vi "ElevFF_CalculateVelocityOnly.vi"(10 "Velocity":dbl, 11 "in ELEV_FF":T1 {"Kg" format="%13.5p"; "Ka" format="%13.5p"; "Kv" format="%13.5p"; "Ks" format="%13.5p"}) -> (3 "FeedForward":dbl)   [LabVIEW 2019, in "Trajectory_Library.lvlib"]
doc: "Calculates the feedforward from the gains and velocity setpoint (acceleration is assumed to be zero).\n \nInputs: \n - ElevFF -- The ElevFF data cluster\n - velocity -- The velocity setpoint.\n\nOutputs:\n - feedforward -- The computed feedforward."
uses:
  Trajectory_Library.lvlib
  ELEV_FF.ctl
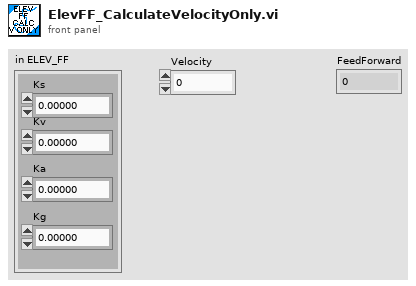
[diagram p1: front panel]
types:
  T1 = typedef "Trajectory_Library.lvlib/ELEV_FF.ctl" = cluster{"Ks":dbl, "Kv":dbl, "Ka":dbl, "Kg":dbl}
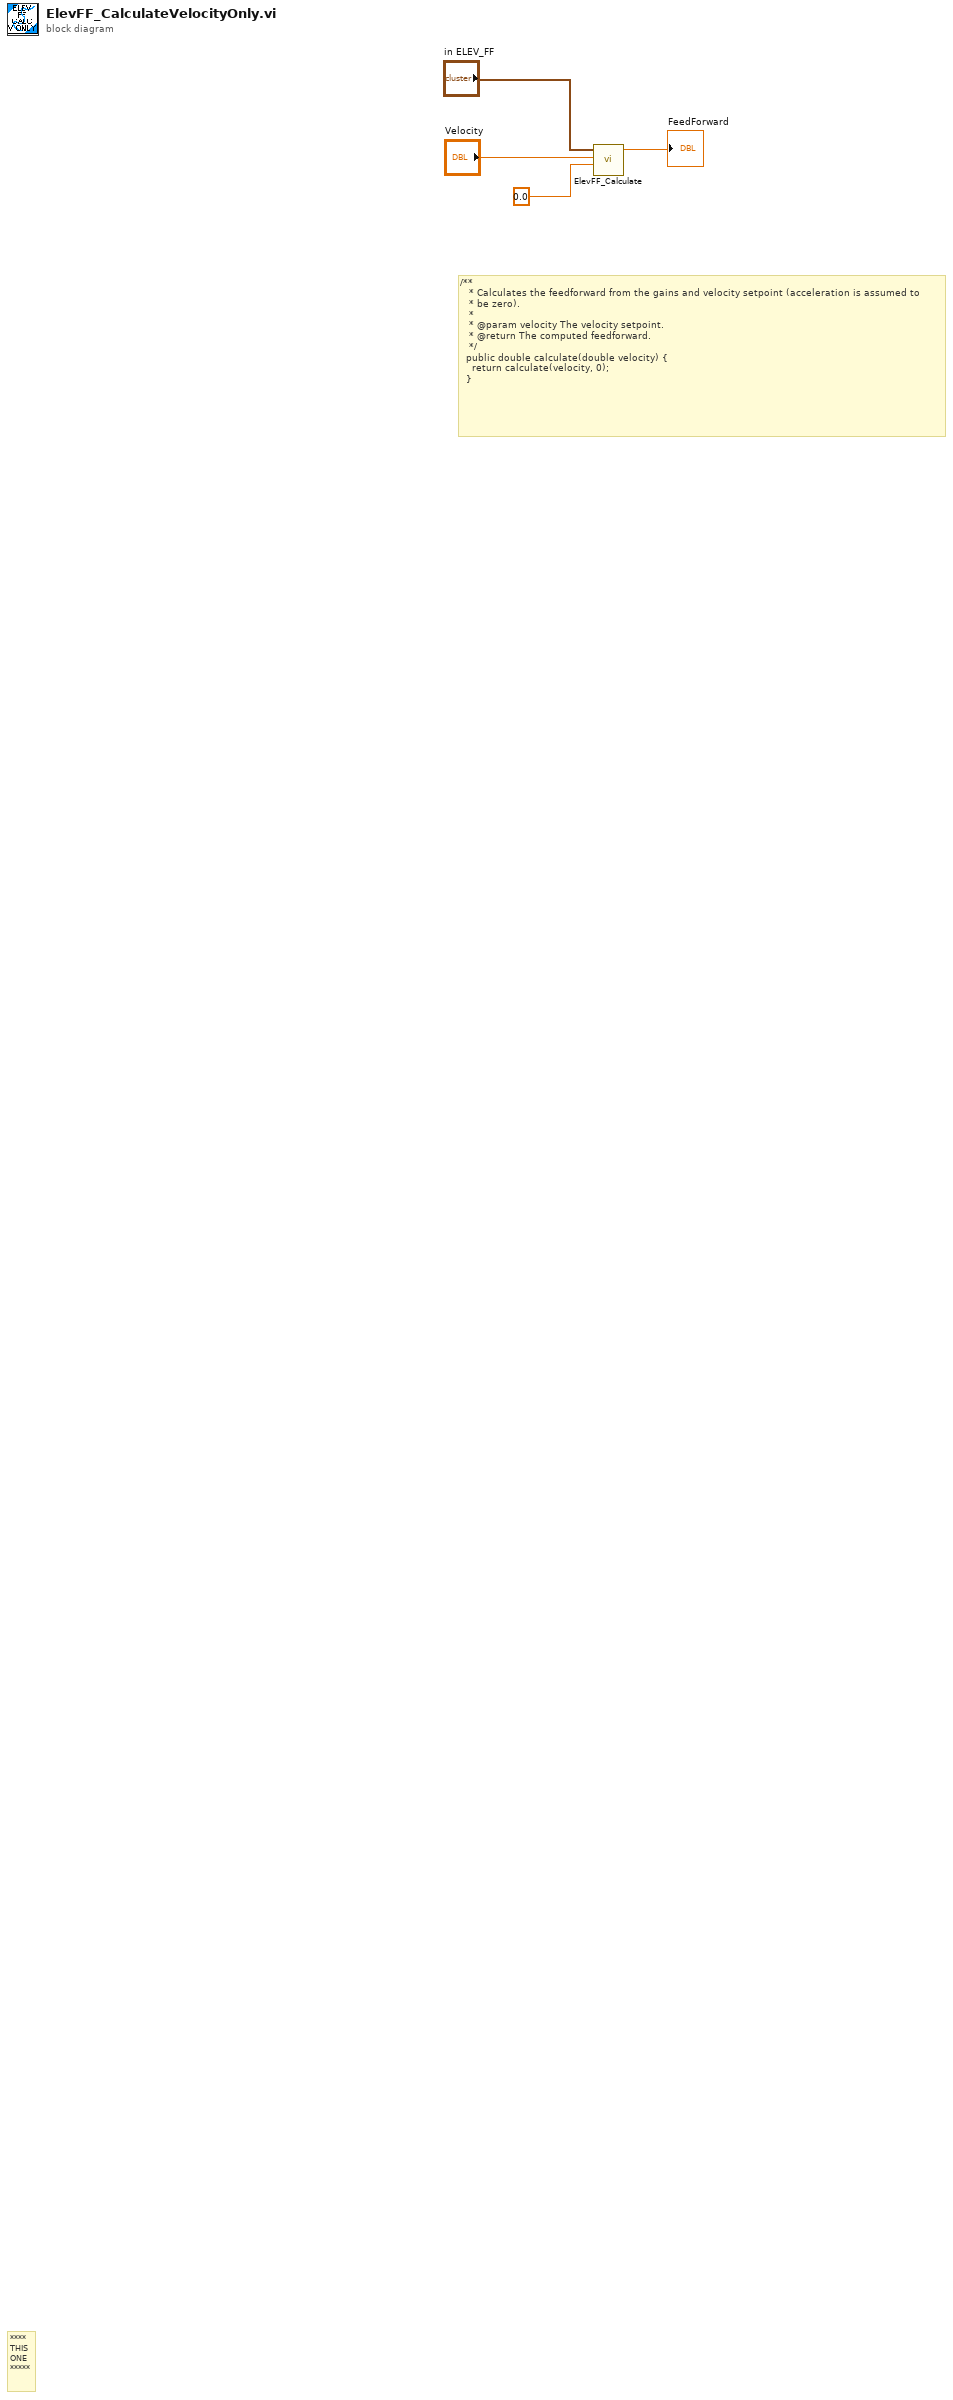
[diagram p0: block diagram]
diagram:
  # "/**\n   * Calculates the feedforward from the gains and velocity setpoint (acceleration is assumed to\n   * be zero).\n   *\n   * @param velocity The velocity setpoint.\n   * @return The computed feedforward.\n   */\n  public double calculate(double velocity) {\n    return calculate(velocity, 0);\n  }"
  # "****\nTHIS\nONE\n*****"
  n1 = call "ElevFF_Calculate.vi"("Accel"=0.0 ("AccelRadPerSecSquared"), "Velocity"="Velocity", "in ELEV_FF"="in ELEV_FF") -> ("FeedForward"=→"FeedForward":dbl)  [unwired: 8 in]
